vi "Get SMO PGSQL Log Paths.vi"(5 "getAll Cluster":variant, 7 "Default Paths":string, 8 "error in (no error)":errorcluster, 11 "Example in":refnum<class "Instrument.LN2.lvclass">) -> (0 "error out":errorcluster, 2 "Paths":string, 3 "Example out":refnum<class "Instrument.LN2.lvclass">)   [LabVIEW 2019, in "Instrument.LN2.lvclass"]
uses:
  Instrument.LN2.lvclass
  Typedefs/Instrument.LN2.getAll--Cluster.ctl
  <userlib>/LevyLab/Instrument Framework/Instrument Types/VSource/Instrument.VSource.lvclass
  <userlib>/LevyLab/LV-Data/LV-Data.PG/LV-Data.PGSQL.lvclass
  <userlib>/LevyLab/LV-Data/LV-Data.PG/API/Write Variable (one-row).vi
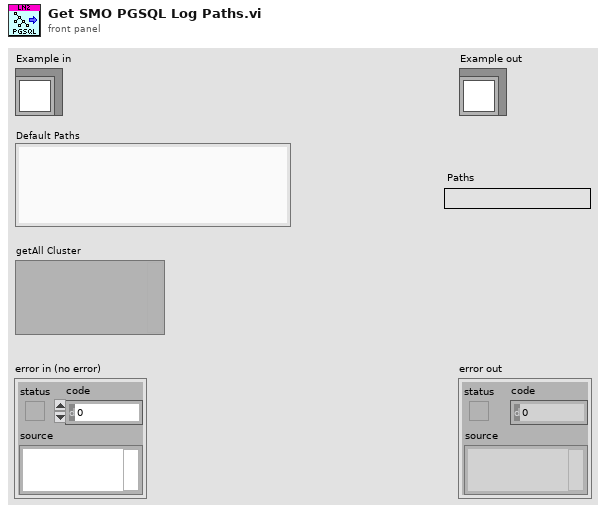
[diagram p1: front panel]
types:
  T1 = typedef "Instrument.LN2.lvclass/Instrument.LN2.getAll--Cluster.ctl" = cluster{"Net Weight(lbs)":dbl, "Gross Weight(lbs) ":dbl, "Tare Weight(lbs) ":dbl, "Empty":dbl}
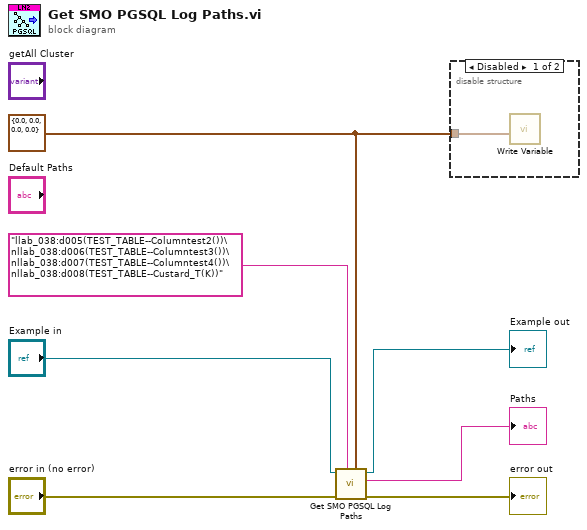
[diagram p0: block diagram]
diagram:
  w1 = T1 {"Net Weight(lbs)"=0.0, "Gross Weight(lbs) "=0.0, "Tare Weight(lbs) "=0.0, "Empty"=0.0} ("getAll")
  n1 = call-parent "Get SMO PGSQL Log Paths.vi"("getAll Cluster"=w1, "Default Paths"="llab_038:d005(TEST_TABLE--Columntest2())\nllab_038:d006(TEST_TABLE--Columntest3())\nllab_038:d007(TEST_TABLE--Columntest4())\nllab_038:d008(TEST_TABLE--Custard_T(K))" ("Paths"), "error in (no error)"="error in (no error)", "Instrument in"="Example in") -> ("error out"=→"error out":errorcluster, "Paths"=→"Paths":string, "Instrument out"=→"Example out":refnum<class "Instrument.LN2.lvclass">)  [unwired: 5 in]
  n2 = disable-structure shown="Disabled" {
    disable-tunnel: w1 -> [w8 _]
    frame Disabled {
      n3 = call-poly <userlib>:"Write Variable.vi"("Data"=w8) -> ()  [unwired: 7 in, 4 out]
    }
    frame Enabled {
    }
  }
